vi "Update Alias pin.vi"(8 "error in (no error)":errorcluster, 9 "New Pin":string, 10 "Alias":string, 11 "Aliases Ref in":T1 format="%.0x") -> (0 "error out":errorcluster, 1 "Replaced":bool, 3 "Aliases Ref out":T1 format="%.0x")   [LabVIEW 2017, in "Switch Scripting.lvlib"]
uses:
  Switch Scripting.lvlib
  <vilib>/NI Veristand/Custom Device API/Custom Device Item Ref.ctl
  <vilib>/NI Veristand/Custom Device API/Set Item Property (String).vi
  <vilib>/NI VeriStand/Custom Device API/Custom Device API.lvlib
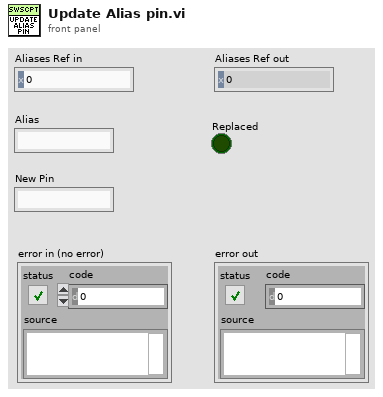
[diagram p1: front panel]
types:
  T1 = typedef "Custom Device API.lvlib/Custom Device Item Ref.ctl" = u64
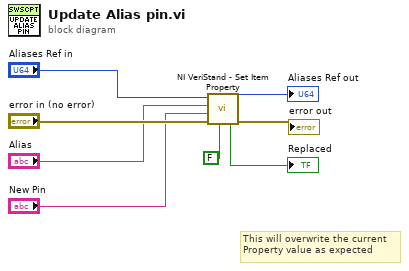
[diagram p0: block diagram]
diagram:
  # "This will overwrite the current\nProperty value as expected"
  n1 = call-poly <vilib>:"NI VeriStand - Set Item Property.vi"("Binary String (T)"=FALSE, "error in (no error)"="error in (no error)", "Value"="New Pin", "Property Name"="Alias", "Item Ref in"="Aliases Ref in") -> ("error out"=→"error out":errorcluster, "Item Ref out"=→"Aliases Ref out":T1, "Replaced"=→"Replaced":bool)  [unwired: 4 in]
